vi "Frame Rate to ms Delay.vi"(9 "Update rate [1/s]":dbl) -> (1 "Wait [ms":i64)   [LabVIEW 2019]
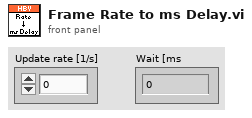
[diagram p1: front panel]
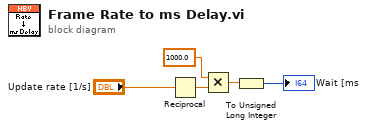
[diagram p0: block diagram]
diagram:
  n1 = Reciprocal(x="Update rate [1/s]") -> (1/x=w3:dbl)
  n2 = Multiply(x=1000.0, y=w3) -> (x*y=w5:dbl)
  n3 = To Unsigned Long Integer(number=w5) -> (unsigned 32bit integer=→"Wait [ms":u32)
